vi "Calc_Portfolio_History_at_Date.vi"(0 "Portfolio en entrée":refnum<class "Portfolio.lvclass"> caption="DNL_LabVIEW Object in", 5 "Date":timestamp, 11 "error in (no error)":errorcluster caption="entrée d'erreur (pas d'erreur)") -> (4 "Portfolio en sortie":refnum<class "Portfolio.lvclass"> caption="DNL_LabVIEW Object out", 8 "Hist Valeur PF":dbl[](graph), 10 "Hist Taux de Perf":dbl[](graph), 13 "Done ?":bool, 15 "error out":errorcluster caption="sortie d'erreur")   [LabVIEW 2012, in "Portfolio.lvclass"]
uses:
  Portfolio.lvclass
  Portfolio.lvclass/Portfolio.ctl
  Stocks Manager/Stock Manager Action.ctl
  Stock/Stock.lvclass/Stock.ctl
  Stock/Stock.lvclass
  Operations/Operations.lvclass
  Exchanges/Exchanges.lvclass
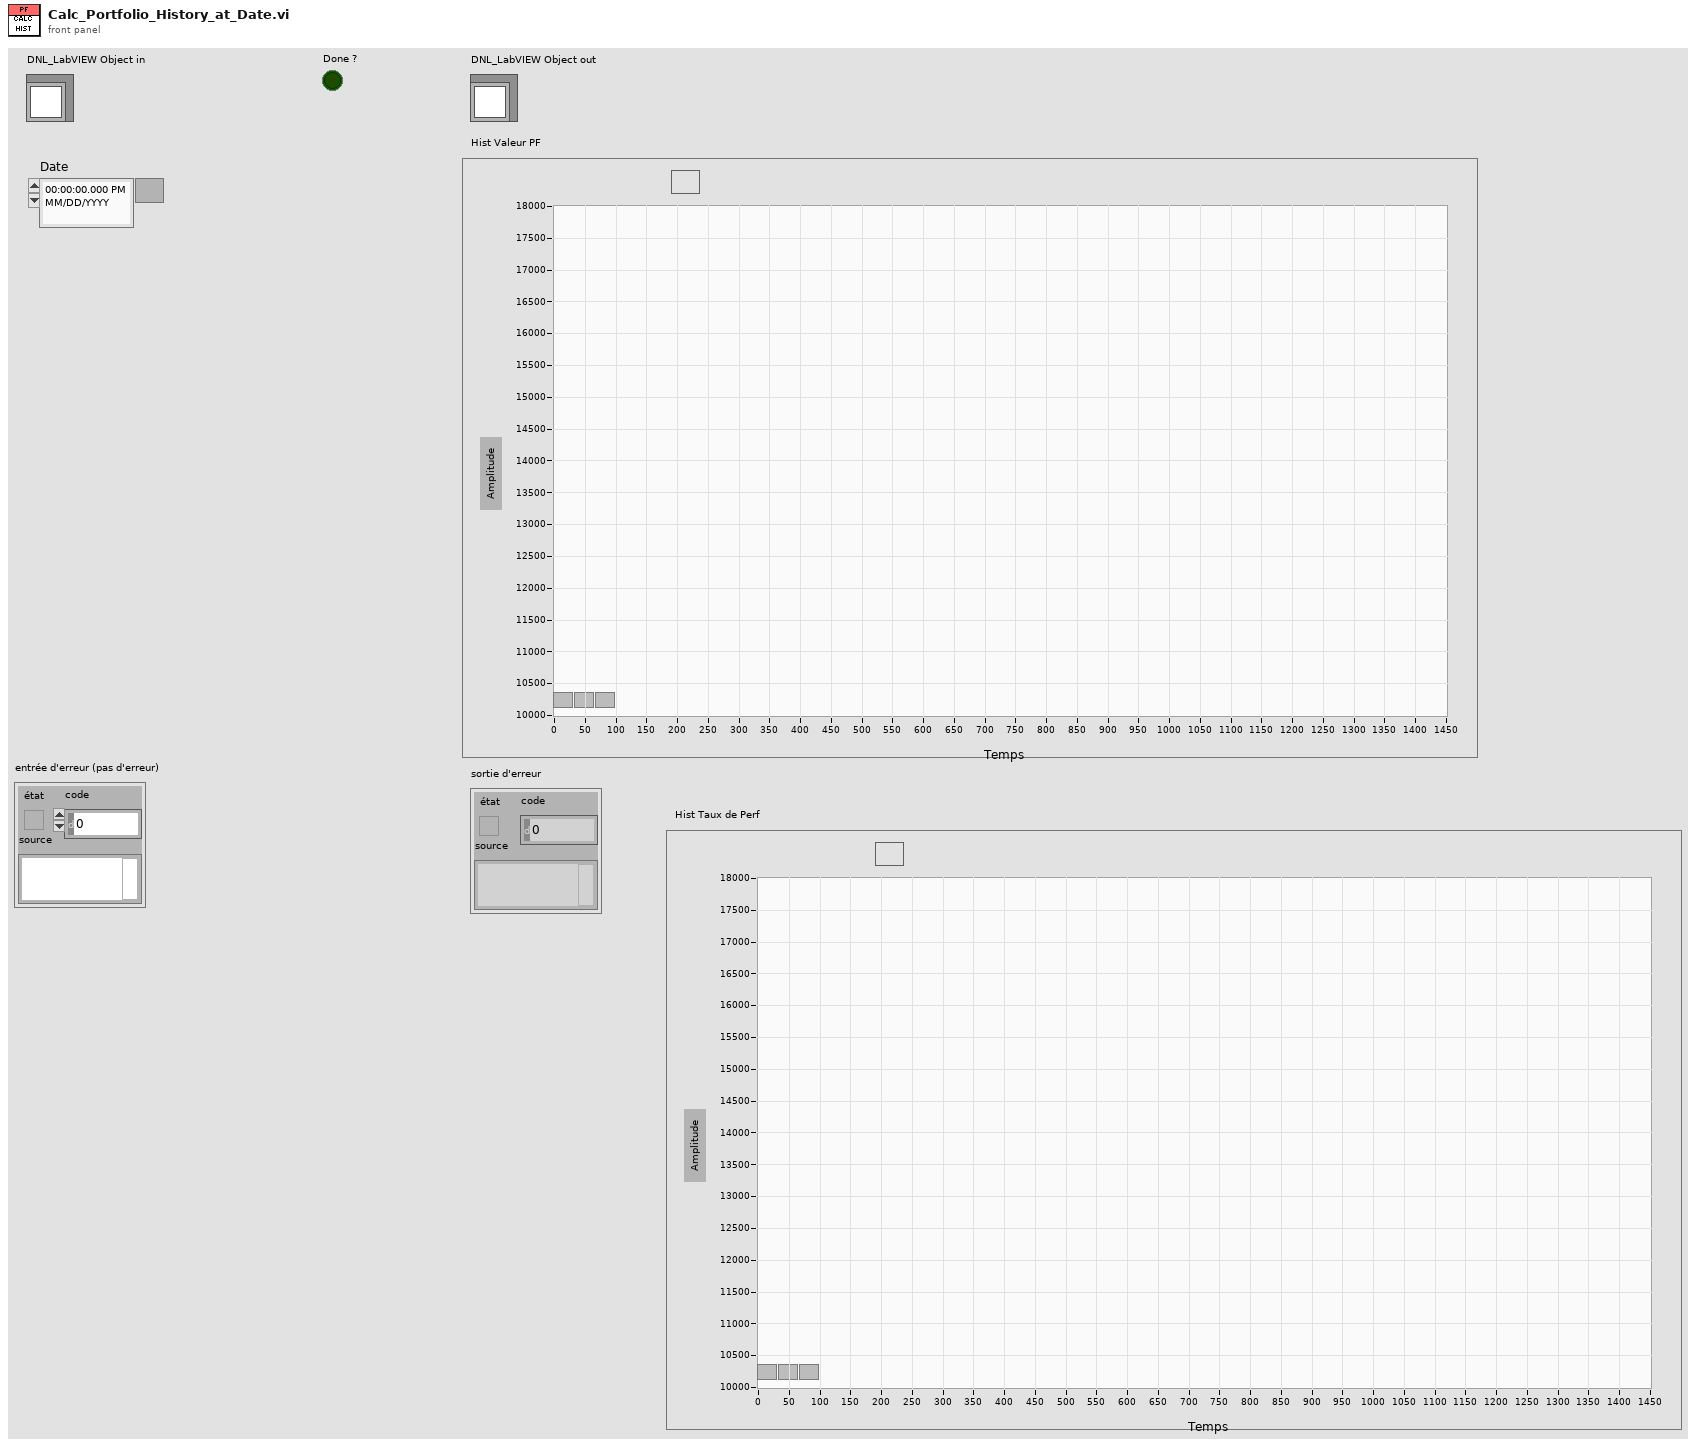
[diagram p1: front panel]
types:
  T1 = typedef "Stock Manager Action.ctl" = enum16{"Get_Stocks", "Load_Stocks", "Find_Stock_From_ISIN", "Find_Stock_From_Label", "Find_Stock_From_Symbol"}
  T2 = typedef "Exchange Parameters.ctl" = cluster{"Date":timestamp, "Exchange Type":T3, "ISIN":string, "Label":string, "Price":dbl, "Qty":dbl, "Currency":T4, "Tax":dbl, "Comment":string, "PRU":dbl}
  T3 = typedef "Exchange.lvclass/Exchange Type Enum.ctl" = enum16{"ACHAT", "VENTE"}
  T4 = typedef "Currencies.ctl" = enum16{"Euro", "Dollar", "Yen", "RIM", "CHF"}
  T5 = typedef "Stock.lvclass/Stock Parameters.ctl" = cluster{"Label":string, "Symbol":string, "Dividend":dbl, "Currency":T4, "ISIN":string, "Symbol_Suffix":string, "Last Price":dbl, "Dividend-Date":string, "Change (%)":dbl}
  T6 = typedef "Operation Parameters.ctl" = cluster{"Date":timestamp, "Operation Type":T7, "Amount":dbl, "Comment":string, "Currency":T4}
  T7 = typedef "Operation Type Enum.ctl" = enum16{"Coupons", "Dépot", "Retrait", "Intérêts", "Taxe"}
  T8 = typedef "Stock_Data.ctl" = cluster{"Date":timestamp, "Open":dbl, "High":dbl, "Low":dbl, "Close":dbl, "Volume":dbl, "Adj Close":dbl}
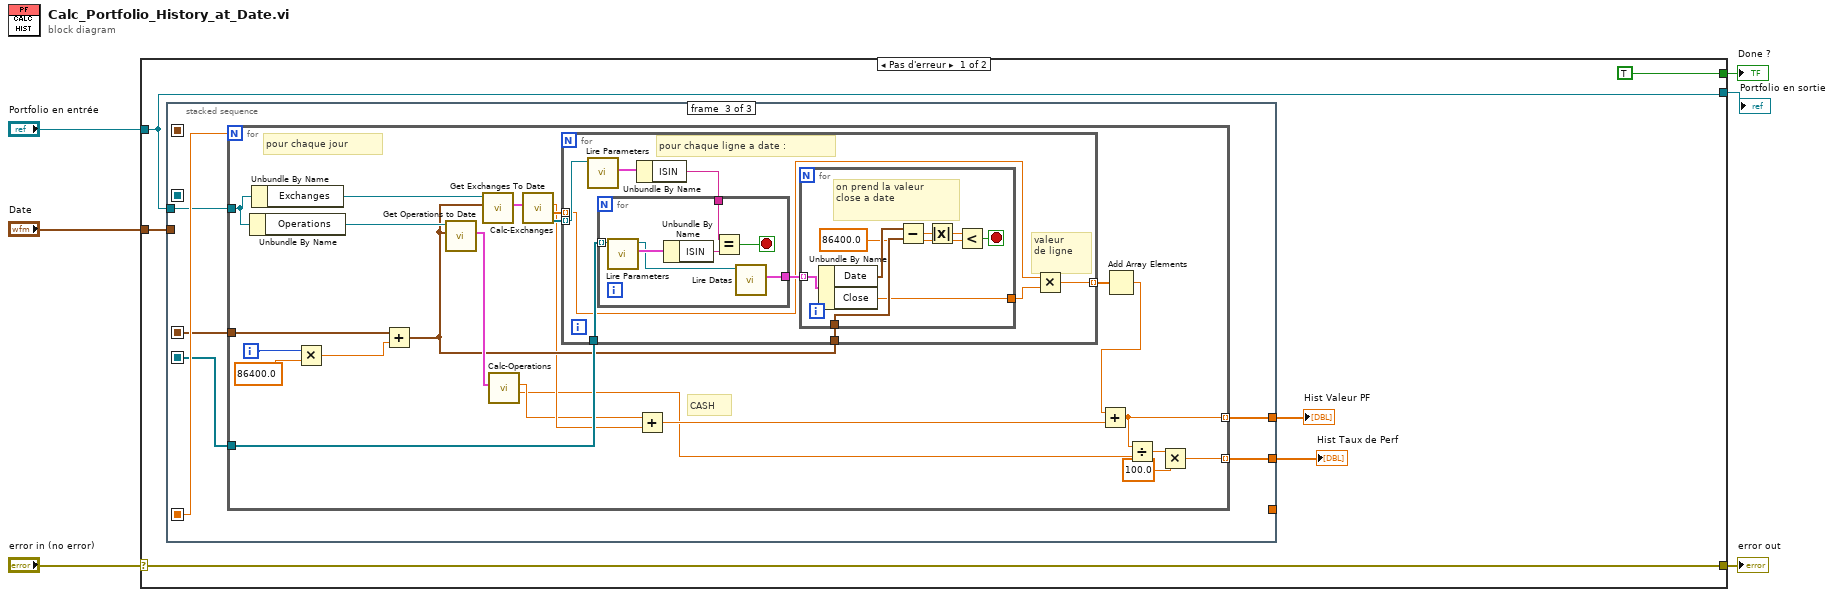
[diagram p0: block diagram]
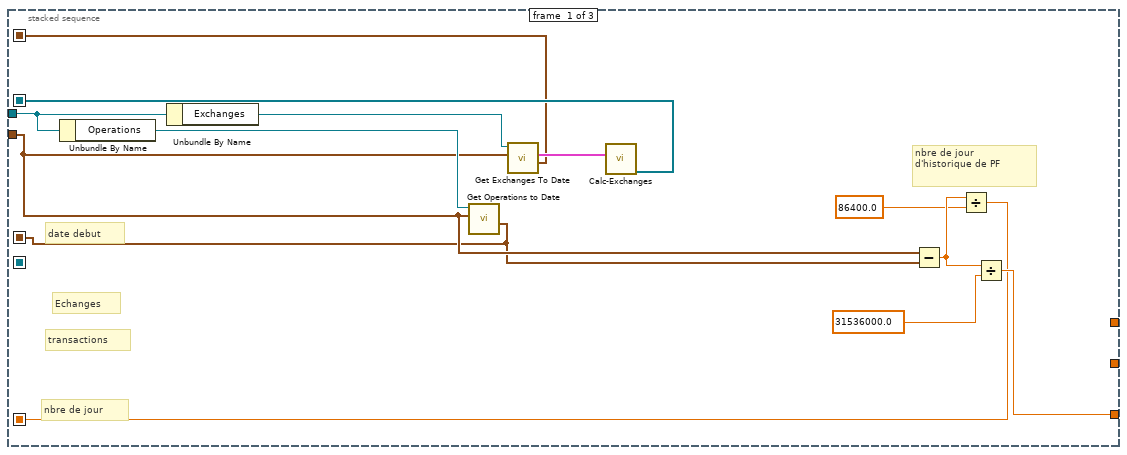
[diagram p2: hidden frame]
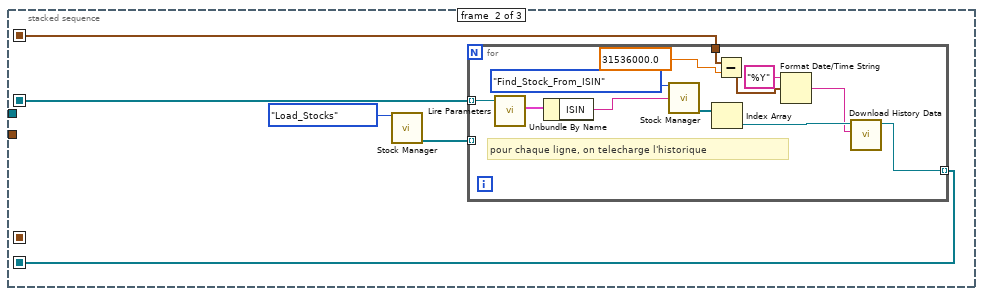
[diagram p3: hidden frame]
diagram:
  n1 = case shown="Pas d'erreur" "error in (no error)" {
    selector: "error in (no error)" -> [w12 w97]
    tunnel: [w12 w97] -> w5
    tunnel: [w9 w96] -> w3
    tunnel: "Portfolio en entrée" -> [w9 w96]
    tunnel: "Date" -> [w11 _]
    tunnel: [TRUE _] -> w1
    frame No Error {
      n2 = stacked-sequence {
        seq-local: [w19 _ _] -> [_ w27 _]
        seq-local: [_ w30 _] -> [_ _ w45]
        seq-local: [w15 _ _] -> [_ _ w48]
        seq-local: [w14 _ _] -> [_ _ w47]
        seq-local: [w13 _ _] -> [_ w26 _]
        tunnel: w9 -> [w21 _ w46]
        tunnel: w11 -> [w20 _ _]
        tunnel: [w24 _ _] -> _
        tunnel: [_ _ w44] -> w8
        tunnel: [_ _ w43] -> w7
        frame #0 {
          # "Echanges"
          # "date debut"
          # "nbre de jour"
          # "nbre de jour\nd'historique de PF"
          # "transactions"
          n3 = Unbundle By Name(w21) -> ("Operations"=w23:refnum<class "Operations.lvclass">)
          n4 = Unbundle By Name(w21) -> ("Exchanges"=w22:refnum<class "Exchanges.lvclass">)
          n5 = call "Get Operations to Date.vi"("Date"=w20, "Operations en entrée"=w23) -> ("Min Date"=w14:timestamp)  [unwired: 6 in, 3 out]
          n6 = call "Get Exchanges To Date.vi"("Date"=w20, "Exchanges en entrée"=w22) -> ("Min Date"=w13:timestamp, "Exchanges to Date"=w18:T2[])  [unwired: 6 in, 2 out]
          n7 = call "Calc-Exchanges.vi"("Exchanges"=w18) -> ("Lignes"=w19:refnum<class "Stock.lvclass">[])  [unwired: 8 in, 2 out]
          n8 = Subtract(x=w20, y=w14) -> (x-y=w17:dbl)
          n9 = Divide(x=w17, y=86400.0) -> (x/y=w15:dbl)
          n10 = Divide(x=w17, y=31536000.0) -> (x/y=w24:dbl)
        }
        frame #1 {
          n11 = call "Stock Manager.vi"("Stock Manager Action"=Stock_Manager_Action."Load_Stocks") -> ("Stocks Found"=w29:refnum<class "Stock.lvclass">[])  [unwired: 12 in, 2 out]
          n12 = for {
            tunnel: w27 -> [w41] mode=indexing
            tunnel: [w36] -> w30 mode=indexing
            tunnel: w29 -> [_] mode=indexing
            tunnel: w26 -> [w33]
            # "pour chaque ligne, on telecharge l'historique"
            n13 = call "Lire Parameters.vi"("Stock en entrée"=w41) -> ("Parameters"=w40:T5)  [unwired: 9 in, 1 out]
            n14 = Unbundle By Name(w40) -> ("ISIN"=w39:string)
            n15 = call "Stock Manager.vi"("Stock Manager Action"=Stock_Manager_Action."Find_Stock_From_ISIN", "String to find (ISIN,Label,Symbol)"=w39) -> ("Stocks Found"=w38:refnum<class "Stock.lvclass">[])  [unwired: 11 in, 2 out]
            n16 = Index Array(array=w38) -> (element=w37:refnum<class "Stock.lvclass">)  [unwired: 1 in]
            n17 = Subtract(x=w33, y=31536000.0) -> (x-y=w31:timestamp)
            n18 = Format Date/Time String(time format string (%c)="%Y" ("chaîne de format de l'heure (%c)"), seconds (now)=w31) -> (date/time string=w34:string)  [unwired: 1 in]
            n19 = call "Download History Data.vi"("Min_Date"=w34, "Share en entrée"=w37) -> ("Share en sortie"=w36:refnum<class "Stock.lvclass">)  [unwired: 6 in, 3 out]
          }
        }
        frame #2 {
          n20 = for {
            N: w48 -> [_]
            tunnel: w47 -> [w71]
            tunnel: w46 -> [w67]
            tunnel: w45 -> [w61]
            tunnel: [w53] -> w44 mode=indexing
            tunnel: [w49] -> w43 mode=indexing
            i -> [w70]
            # "CASH"
            # "pour chaque jour"
            n21 = Unbundle By Name(w67) -> ("Operations"=w65:refnum<class "Operations.lvclass">)
            n22 = Unbundle By Name(w67) -> ("Exchanges"=w66:refnum<class "Exchanges.lvclass">)
            n23 = Multiply(x=w70, y=86400.0) -> (x*y=w68:dbl)
            n24 = Add(x=w71, y=w68) -> (x+y=w60:timestamp)
            n25 = call "Get Operations to Date.vi"("Date"=w60, "Operations en entrée"=w65) -> ("Operations Found at Date"=w63:T6[])  [unwired: 6 in, 3 out]
            n26 = call "Get Exchanges To Date.vi"("Date"=w60, "Exchanges en entrée"=w66) -> ("Exchanges to Date"=w64:T2[])  [unwired: 6 in, 3 out]
            n27 = call "Calc-Operations.vi"("Operations"=w63) -> ("Investissement"=w52:dbl, "Total OP"=w55:dbl)  [unwired: 9 in]
            n28 = call "Calc-Exchanges.vi"("Exchanges"=w64) -> ("Lignes"=w62:refnum<class "Stock.lvclass">[], "Qtés restante par ligne"=w59:dbl[], "Total"=w56:dbl)  [unwired: 8 in]
            n29 = for {
              tunnel: w62 -> [w79] mode=indexing
              tunnel: w61 -> [w77]
              tunnel: w60 -> [w75]
              tunnel: w59 -> [w74] mode=indexing
              tunnel: [w73] -> w58 mode=indexing
              # "valeur\nde ligne"
              # "pour chaque ligne a date :"
              n30 = call "Lire Parameters.vi"("Stock en entrée"=w79) -> ("Parameters"=w80:T5)  [unwired: 9 in, 1 out]
              n31 = Unbundle By Name(w80) -> ("ISIN"=w78:string)
              n32 = for {
                tunnel: w78 -> [w94]
                tunnel: w77 -> [w92] mode=indexing
                tunnel: [w89] -> w76
                stop <- w91 stop-if-true
                n33 = call "Lire Parameters.vi"("Stock en entrée"=w92) -> ("Parameters"=w95:T5, "Stock en sortie"=w90:refnum<class "Stock.lvclass">)  [unwired: 9 in]
                n34 = Unbundle By Name(w95) -> ("ISIN"=w93:string)
                n35 = Equal?(x=w94, y=w93) -> (x = y?=w91:bool)
                n36 = call "Lire Datas.vi"("Share en entrée"=w90) -> ("Datas"=w89:T8[])  [unwired: 8 in, 2 out]
              }
              n37 = for {
                tunnel: w76 -> [w88] mode=indexing
                tunnel: w75 -> [w86]
                tunnel: [w81] -> w72
                stop <- w82 stop-if-true
                # "on prend la valeur\nclose a date"
                n38 = Unbundle By Name(w88) -> ("Date"=w87:timestamp, "Close"=w81:dbl)
                n39 = Subtract(x=w87, y=w86) -> (x-y=w85:dbl)
                n40 = Absolute Value(x=w85) -> (abs(x)=w84:dbl)
                n41 = Less?(x=w84, y=86400.0) -> (x < y?=w82:bool)
              }
              n42 = Multiply(x=w74, y=w72) -> (x*y=w73:dbl)
            }
            n43 = Add(x=w55, y=w56) -> (x+y=w54:dbl)
            n44 = Add Array Elements(numeric array=w58) -> (sum=w57:dbl)
            n45 = Add(x=w57, y=w54) -> (x+y=w53:dbl)
            n46 = Divide(x=w53, y=w52) -> (x/y=w51:dbl)
            n47 = Multiply(x=w51, y=100.0) -> (x*y=w49:dbl)
          }
        }
      }
      "Hist Valeur PF" <- w8
      "Hist Taux de Perf" <- w7
    }
    frame Error {
    }
  }
  "error out" <- w5
  "Portfolio en sortie" <- w3
  "Done ?" <- w1
